vi "fesa lamp.vi"(2 "FESA values":u16[](array[numeric])) -> (0 "lamp1":u16[](array[numeric]), 1 "lamp2":u16[](array[numeric]), 3 "lamp10":u16[](array[numeric]), 4 "lamp9":u16[](array[numeric]), 5 "lamp3":u16[](array[numeric]), 6 "lamp4":u16[](array[numeric]), 7 "lamp5":u16[](array[numeric]), 8 "lamp8":u16[](array[numeric]), 9 "lamp6":u16[](array[numeric]), 10 "lamp7":u16[](array[numeric]))   [LabVIEW 2017]
panel:
  out "Array":u16[][](array[numeric])
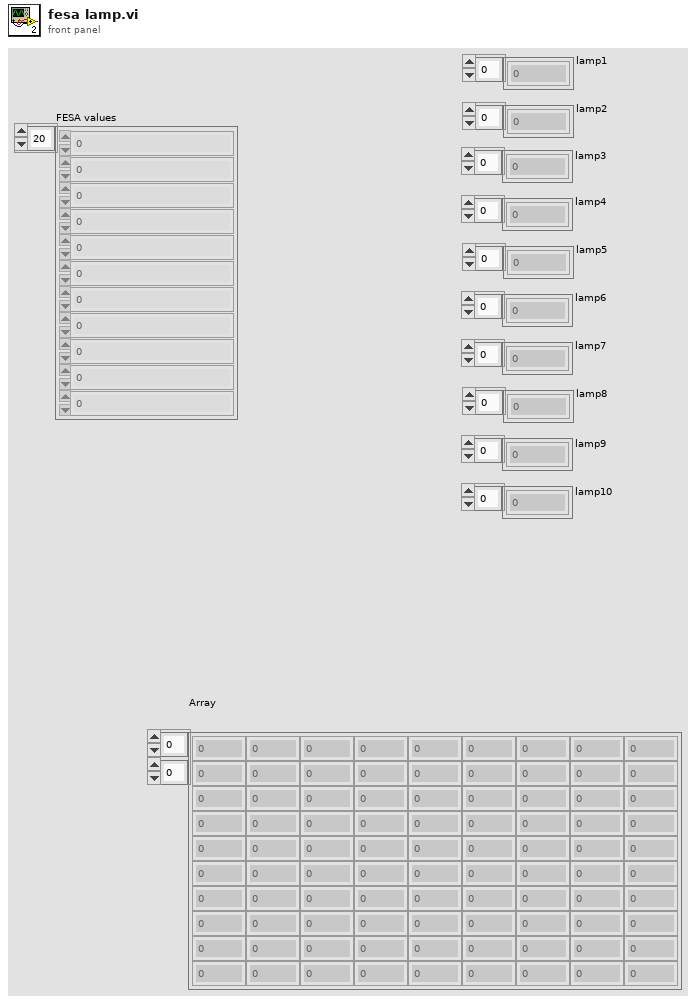
[diagram p1: front panel]
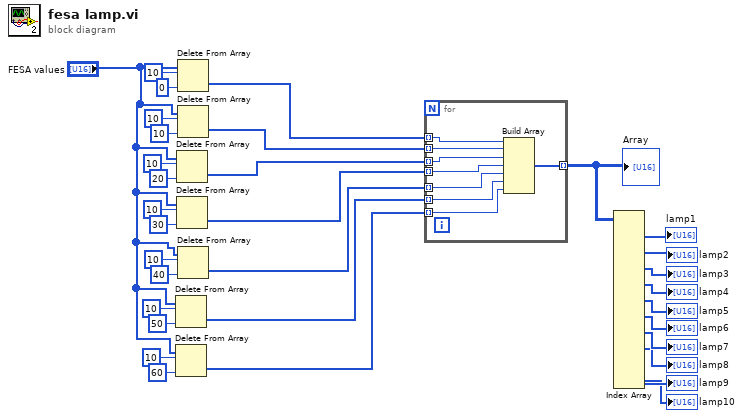
[diagram p0: block diagram]
diagram:
  n1 = Delete From Array(array="FESA values", length=10, index=50) -> (deleted portion=w13:u16[])  [unwired: 1 out]
  n2 = Delete From Array(array="FESA values", length=10, index=60) -> (deleted portion=w12:u16[])  [unwired: 1 out]
  n3 = Delete From Array(array="FESA values", length=10, index=20) -> (deleted portion=w16:u16[])  [unwired: 1 out]
  n4 = Delete From Array(array="FESA values", length=10, index=30) -> (deleted portion=w15:u16[])  [unwired: 1 out]
  n5 = Delete From Array(array="FESA values", length=10, index=0) -> (deleted portion=w18:u16[])  [unwired: 1 out]
  n6 = Delete From Array(array="FESA values", length=10, index=10) -> (deleted portion=w17:u16[])  [unwired: 1 out]
  n7 = Delete From Array(array="FESA values", length=10, index=40) -> (deleted portion=w14:u16[])  [unwired: 1 out]
  n8 = for {
    tunnel: w18 -> [w41] mode=indexing
    tunnel: w17 -> [w40] mode=indexing
    tunnel: w16 -> [w39] mode=indexing
    tunnel: w15 -> [w38] mode=indexing
    tunnel: w14 -> [w37] mode=indexing
    tunnel: w13 -> [w36] mode=indexing
    tunnel: w12 -> [w35] mode=indexing
    tunnel: [w34] -> w11 mode=indexing
    n9 = Build Array(w41, w40, w39, w38, w37, w36, w35) -> (w34:u16[])
  }
  "Array" <- w11
  n10 = Index Array(array=w11) -> (element #1=→"lamp1":u16[], element #2=→"lamp2":u16[], element #3=→"lamp3":u16[], element #4=→"lamp4":u16[], element #5=→"lamp5":u16[], element #6=→"lamp6":u16[], element #7=→"lamp7":u16[], element #8=→"lamp8":u16[], element #9=→"lamp9":u16[], element #10=→"lamp10":u16[])  [unwired: 20 in]
